vi "Create CVT Tag.vi"(8 "error in (no error)":errorcluster) -> (0 "error out":errorcluster)   [LabVIEW 2016, in "CVT.lvlib"]
uses:
  CVT.lvlib
  Support Libraries/Current Value Table/Type Defs/File Format.ctl
  Support Libraries/Current Value Table/Type Defs/Single Tag.ctl
  Support Libraries/Current Value Table/Type Defs/Data Types.ctl
  Support Libraries/Current Value Table/Type Defs/Tag Grouping set.ctl
  Support Libraries/Current Value Table/Current Value Table.lvlib
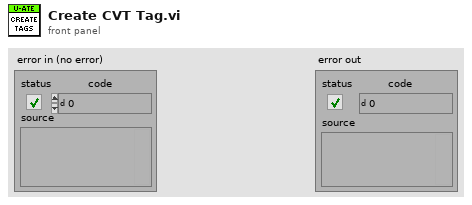
[diagram p1: front panel]
types:
  T1 = typedef "CVT.lvlib/Current Value Table.lvlib/File Format.ctl" = cluster{"Tags":T2[], "Group Listings":T4[]}
  T2 = typedef "CVT.lvlib/Current Value Table.lvlib/Single Tag.ctl" = cluster{"Data Type":T3, "Name":string, "Value":string, "Description":string}
  T3 = typedef "CVT.lvlib/Current Value Table.lvlib/Data Types.ctl" = enum16{"Double", "Single", "I64", "I32", "I16", "I8", "U64", "U32", "U16", "U8", "String", "Boolean", "Array of U8", "Array of U16", "Array of U32", "Array of U64", "Array of I64", "Array of I32", "Array of I16", "Array of I8", "Array of Double", "Array of Single", "Array of Boolean", "Array of String"}
  T4 = typedef "CVT.lvlib/Current Value Table.lvlib/Tag Grouping set.ctl" = cluster{"Group":string, "Tag Names":string[]}
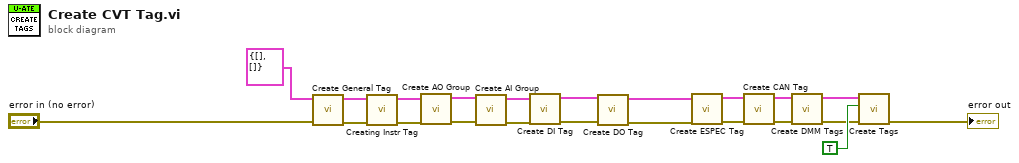
[diagram p0: block diagram]
diagram:
  n1 = call "Create General Tag.vi"("error in (no error)"="error in (no error)", "CVT Tags to Create"=T1 {"Tags"=[], "Group Listings"=[]}) -> ("error out"=w16:errorcluster, "CVT Tags to Create"=w17:T1)  [unwired: 8 in]
  n2 = call "Creating Instr Tag.vi"("error in (no error)"=w16, "CVT Tags to Create"=w17) -> ("error out"=w15:errorcluster, "CVT Tags to Create 2"=w14:T1)  [unwired: 8 in]
  n3 = call "Create AO Group.vi"("error in (no error)"=w15, "CVT Tags to Create"=w14) -> ("error out"=w21:errorcluster, "CVT Tags to Create 2"=w20:T1)  [unwired: 8 in]
  n4 = call "Create AI Group.vi"("error in (no error)"=w21, "CVT Tags to Create"=w20) -> ("error out"=w19:errorcluster, "CVT Tags to Create 2"=w18:T1)  [unwired: 8 in]
  n5 = call "Create DI Tag.vi"("error in (no error)"=w19, "CVT Tags to Create"=w18) -> ("error out"=w2:errorcluster, "CVT Tags to Create 2"=w4:T1)  [unwired: 8 in]
  n6 = call "Create DO Tag.vi"("error in (no error)"=w2, "CVT Tags to Create"=w4) -> ("error out"=w1:errorcluster, "CVT Tags to Create"=w3:T1)  [unwired: 8 in]
  n7 = call "Create ESPEC Tag.vi"("error in (no error)"=w1, "CVT Tags to Create"=w3) -> ("error out"=w13:errorcluster, "CVT Tags to Create 2"=w12:T1)  [unwired: 8 in]
  n8 = call "Create CAN Tag.vi"("error in (no error)"=w13, "CVT Tags to Create"=w12) -> ("error out"=w8:errorcluster, "CVT Tags to Create 2"=w7:T1)  [unwired: 8 in]
  n9 = call "Create DMM Tags.vi"("error in (no error)"=w8, "CVT Tags to Create"=w7) -> ("error out"=w5:errorcluster, "CVT Tags to Create"=w6:T1)  [unwired: 8 in]
  n10 = call "Create Tags.vi"("error in (no error)"=w5, "Clear Table? (F)"=TRUE, "CVT Tags to Create"=w6) -> ("error out"=→"error out":errorcluster)  [unwired: 8 in]
